vi "System_Read TagBus_DELETEME.vi"(11 "System in":refnum<class "System.lvclass">) -> (2 "TagBus.lvclass":refnum<class "TagBus.lvclass">, 3 "System out":refnum<class "System.lvclass">)   [LabVIEW 2015]
uses:
  System.lvclass
  TagBus/TagBus.lvclass
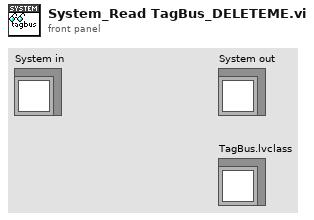
[diagram p1: front panel]
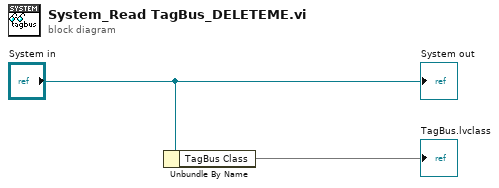
[diagram p0: block diagram]
diagram:
  n1 = Unbundle By Name("System in") -> ("TagBus Class"=→"TagBus.lvclass")
  "System out" <- "System in"
